vi "Read Config from File.vi"(8 "error in (no error)":errorcluster) -> (0 "error out":errorcluster, 3 "System Parameters":T1={"Optical /HW Parameters"={"Focal Length [mm]"=1.0, "Scan Lens EFL[mm]"=0.0, "Tube Lens EFL[mm]"=0.0, "Galvo V Range (+/-)"=0.0, "Galvo Max Half Angle [Deg]"=0.0, "Max Galvo Range[%]"=0.0}, "Vibratome"={"Z Bottom [mm]"=0.0, "Pre Cut Dwell [s]"=0.0, "Blade Frequency [RPM]"=0, "Slice Speed [mm/s]"=0.0, "Post Cut Dwell [s]"=0.0, "Ramp Time [s]"=0.0, "Start X [mm]"=0.0, "Start Y [mm]"=0.0, "Slice Length [mm]"=0.0, "Slice Axis"=enum."Y Axis", "Controller VISA Ref"="COM4"}, "Table Stages"={"X Stage"={"Position"=0.0, "Is.Enabled?"=FALSE, "Is.Connected?"=FALSE, "Device SN"="45876539", "AccelerationMaximum"=0.0, "VelocityMaximum"=0.0, "Acceleration"=0.0, "Velocity"=0.0, "waitTimeout (ms)"=0, "Model"=enum."None", "Is.Homed?"=FALSE}, "Y Stage"={"Position"=0.0, "Is.Enabled?"=FALSE, "Is.Connected?"=FALSE, "Device SN"="45876539", "AccelerationMaximum"=0.0, "VelocityMaximum"=0.0, "Acceleration"=0.0, "Velocity"=0.0, "waitTimeout (ms)"=0, "Model"=enum."None", "Is.Homed?"=FALSE}, "Z Stage"={"Position"=0.0, "Is.Enabled?"=FALSE, "Is.Connected?"=FALSE, "Device SN"="45876539", "AccelerationMaximum"=0.0, "VelocityMaximum"=0.0, "Acceleration"=0.0, "Velocity"=0.0, "waitTimeout (ms)"=0, "Model"=enum."None", "Is.Homed?"=FALSE}}, "Imaging Parameter"={"Pixel Dwell Time [ms]"=1.0, "XY Center [um]"={"X"=1.0, "Y"=1.0}, "Zoom Factor"=1.0, "Display Channel"=enum."Channel A", "XY Image Resolution"=enum."256 x 256", "Custom"=FALSE, "Custom Size"={"X"=1, "Y"=1}, "Averaging"={"A Frame Ave."=1, "B Frame Ave."=1, "C Frame Ave. "=1}}} {"Imaging Parameter"."Custom Size"."Y" min=1 max=30 step=1; "Imaging Parameter"."Custom Size"."X" min=1 max=30 step=1; "Imaging Parameter"."XY Center [um]"."Y" min=1.0 max=30.0 step=1.0; "Imaging Parameter"."XY Center [um]"."X" min=1.0 max=30.0 step=1.0; "Imaging Parameter"."Averaging"."C Frame Ave." min=1 max=30 step=1; "Imaging Parameter"."Averaging"."B Frame Ave." min=1 max=30 step=1; "Imaging Parameter"."Averaging"."A Frame Ave." min=1 max=30 step=1; "Imaging Parameter"."Zoom Factor" min=1.0 max=10.0 step=0.1 scale=1.0..30.0; "Imaging Parameter"."Pixel Dwell Time [ms]" min=0.0 max=10.0 step=0.01})   [LabVIEW 2017]
uses:
  Controls/System Parameters.ctl
  Hardware/Table Stage/Controls/Translation Stage Cluster.ctl
  Controls/Translation Stage Types.ctl
  <vilib>/Utility/config.llb/NI_LVConfig.lvlib
panel:
  # "X"
  # "X"
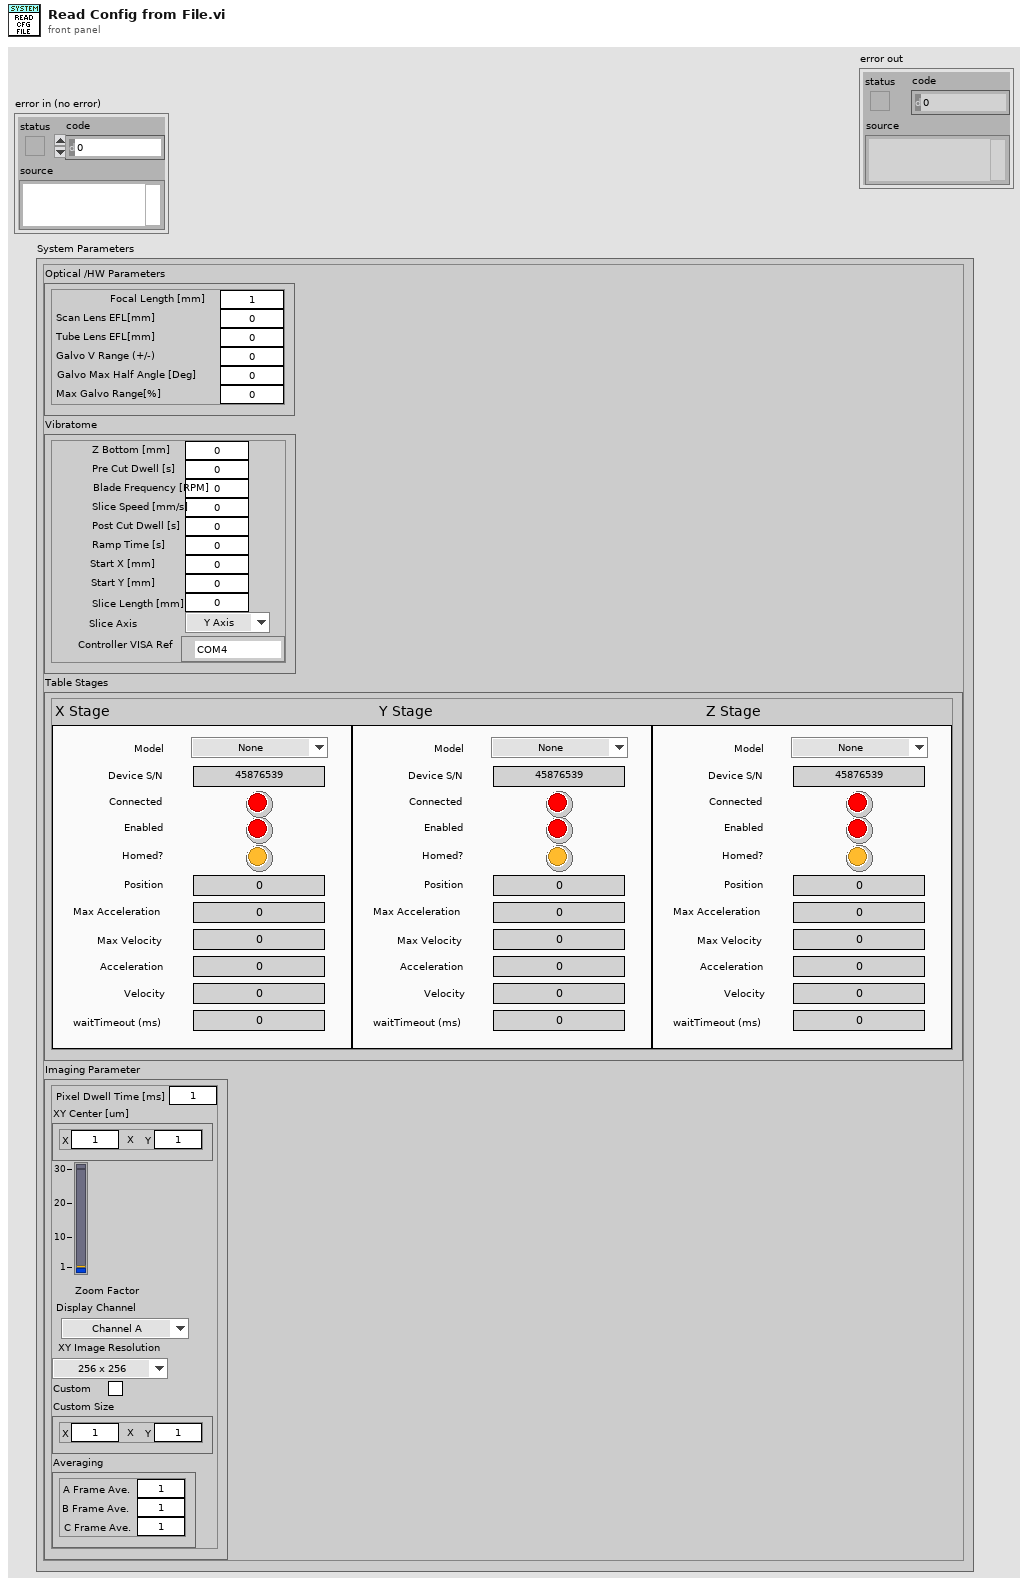
[diagram p1: front panel]
types:
  T1 = typedef "System Parameters.ctl" = cluster{"Optical /HW Parameters":cluster{"Focal Length [mm]":dbl, "Scan Lens EFL[mm]":dbl, "Tube Lens EFL[mm]":dbl, "Galvo V Range (+/-)":dbl, "Galvo Max Half Angle [Deg]":dbl, "Max Galvo Range[%]":dbl}, "Vibratome":cluster{"Z Bottom [mm]":dbl, "Pre Cut Dwell [s]":dbl, "Blade Frequency [RPM]":u16, "Slice Speed [mm/s]":dbl, "Post Cut Dwell [s]":dbl, "Ramp Time [s]":dbl, "Start X [mm]":dbl, "Start Y [mm]":dbl, "Slice Length [mm]":dbl, "Slice Axis":enum16{"X Axis", "Y Axis", "Z Axis"}, "Controller VISA Ref":refnum<visa-resource-name>}, "Table Stages":cluster{"X Stage":T2, "Y Stage":T2, "Z Stage":T2}, "Imaging Parameter":cluster{"Pixel Dwell Time [ms]":dbl, "XY Center [um]":cluster{"X":dbl, "Y":dbl}, "Zoom Factor":dbl, "Display Channel":enum16{"Channel A", "Channel B", "Channel A and B"}, "XY Image Resolution":enum16{"32 x 32", "64 x 64", "128 x 128", "256 x 256", "512 x 512", "1024 x 1024", "2048 x 2048"}, "Custom":bool, "Custom Size":cluster{"X":u16, "Y":u16}, "Averaging":cluster{"A Frame Ave.":u8, "B Frame Ave.":u8, "C Frame Ave. ":u8}}}
  T2 = typedef "Translation Stage Cluster.ctl" = cluster{"Position":dbl, "Is.Enabled?":bool, "Is.Connected?":bool, "Device SN":string, "AccelerationMaximum":dbl, "VelocityMaximum":dbl, "Acceleration":dbl, "Velocity":dbl, "waitTimeout (ms)":i32, "Model":T3, "Is.Homed?":bool}
  T3 = typedef "Translation Stage Types.ctl" = enum16{"None", "Thorlabs LTS", "Thorlabs MLJ"}
  T4 = typedef "NI_LVConfig.lvlib/Config Data RefNum.ctl" = refnum<k1>
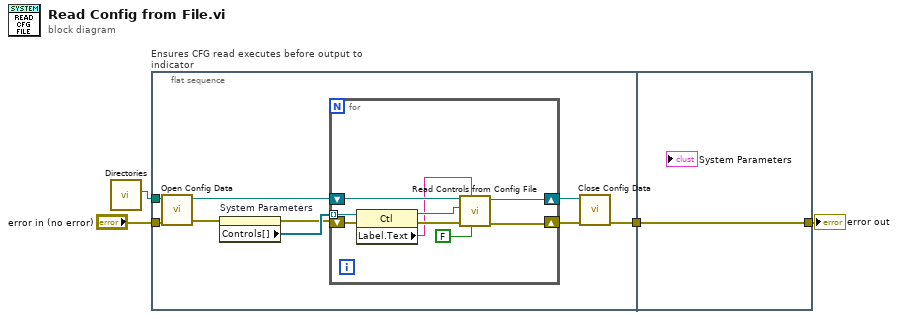
[diagram p0: block diagram]
diagram:
  n1 = call "Directories.vi"() -> ("Config.ini Path"=w2:path)  [unwired: 10 in, 1 out]
  n2 = flat-sequence "Ensures CFG read executes before output to indicator" {
    tunnel: "error in (no error)" -> [w13]
    tunnel: w2 -> [w11]
    tunnel: [w12] -> w1
    tunnel: [w23] -> w3
    tunnel: w1 -> [w23]
    frame #0 {
      n3 = call <vilib>:"Open Config Data.vi"("error in (no error)"=w13, "configuration file path"=w11) -> ("error out"=w5:errorcluster, "refnum"=w8:T4)  [unwired: 7 in, 1 out]
      n4 = property on="System Parameters" class="Clust"(error in=w5) -> (error out=w6:errorcluster, "Controls[]"=w10:refnum<vi>[])  [unwired: 1 in, 1 out]
      n5 = for {
        tunnel: w10 -> [w22] mode=indexing
        shift-right: [w18] -> w9
        shift-left: w6 -> [w21]
        shift-right: [w14] -> w7
        shift-left: w8 -> [w17]
        n6 = property class="Ctl"(reference=w22, error in=w21) -> (reference out=w16:refnum<vi>, error out=w19:errorcluster, "Label.Text"=w15:string)
        n7 = call "Read Controls from Config File.vi"("Child?"=FALSE, "section"=w15, "Error In"=w19, "Ctl Refnum"=w16, "refnum"=w17) -> ("Error Out"=w18:errorcluster, "refnum out"=w14:T4)  [unwired: 5 in]
      }
      n8 = call <vilib>:"Close Config Data.vi"("error in (no error)"=w9, "refnum"=w7) -> ("error out"=w12:errorcluster)  [unwired: 8 in, 1 out]
    }
    frame #1 {
    }
  }
  "error out" <- w3
